vi "Number of Plots Write.vi"(4 "error in (no error)":errorcluster, 5 "Value":i32, 6 "Container State":T2, 7 "Display State In":T1 {"Time_data" format="%<%.3X>T"}) -> (0 "error out":errorcluster, 3 "Display State Out":T1 {"Time_data" format="%<%.3X>T"})   [LabVIEW 2015, in "Two Axis.xctl"]
uses:
  Two Axis.xctl
  <vilib>/_xctls/Container State.ctl
  Two Axis State.ctl
  <vilib>/_xctls/XControlSupport.lvlib
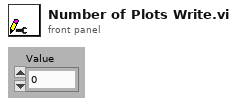
[diagram p1: front panel]
types:
  T1 = typedef "Two Axis.xctl/Two Axis State.ctl" = cluster{"History":i32, "Time_data":timestamp[], "Data_Out":sgl[][], "NumPlots":i32, "LegElem":i32, "Plot Details":cluster{"Name":string, "Line Width":u8, "Line Style":u8, "Color":u32}[], "Y-Axis Labels":string[], "Title":string, "data_only?":bool}
  T2 = typedef "XControlSupport.lvlib/Container State.ctl" = cluster{"Indicator?":bool, "Run Mode?":bool, " Refnum":refnum<vi>}
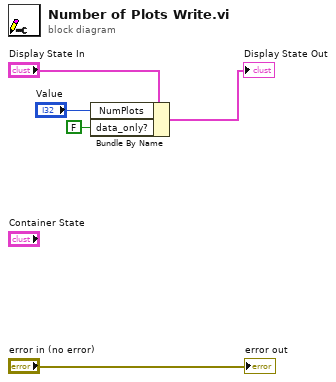
[diagram p0: block diagram]
diagram:
  n1 = Bundle By Name(cluster="Display State In", "NumPlots"="Value", "data_only?"=FALSE) -> (→"Display State Out":T1)
  "error out" <- "error in (no error)"
